vi "Read Com_Set.vi"(8 "error in (no error)":errorcluster, 11 "RS232 in":refnum<class "RS232.lvclass">) -> (0 "error out":errorcluster, 2 "Com_Set":T1, 3 "RS232 out":refnum<class "RS232.lvclass">)   [LabVIEW 2019, in "RS232.lvclass"]
uses:
  RS232.lvclass
  SettingCtrl.ctl
  RS232.lvclass/RS232.ctl
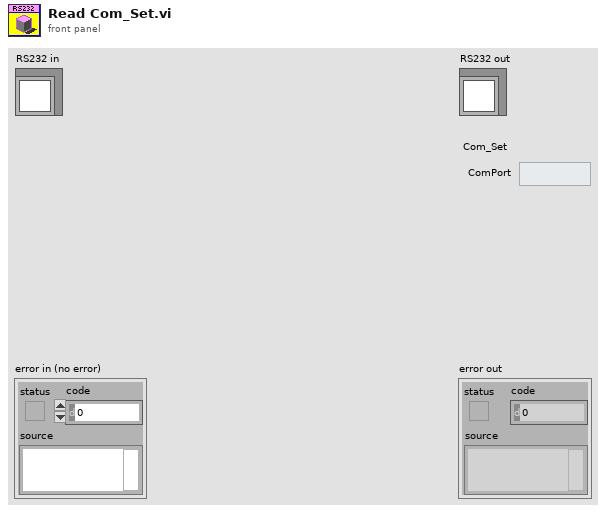
[diagram p1: front panel]
types:
  T1 = typedef "RS232.lvclass/SettingCtrl.ctl" = cluster{"ComPort":string}
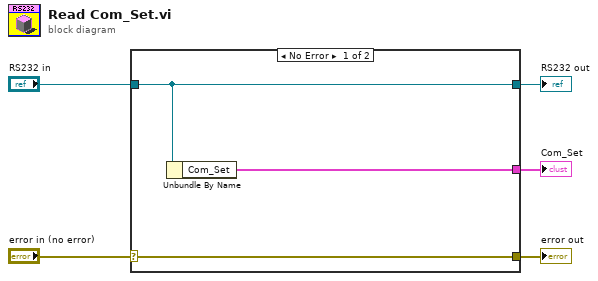
[diagram p0: block diagram]
diagram:
  n1 = case shown="No Error" "error in (no error)" {
    selector: "error in (no error)" -> [w8 w9]
    tunnel: [w8 w9] -> w4
    tunnel: [w7 w10] -> w2
    tunnel: "RS232 in" -> [w7 w10]
    tunnel: [w6 _] -> w1
    frame No Error {
      n2 = Unbundle By Name(w7) -> ("Com_Set"=w6:T1)
    }
    frame Error {
    }
  }
  "error out" <- w4
  "RS232 out" <- w2
  "Com_Set" <- w1
